vi "Create_Trajectory_Make_Trajectory.vi"(6 "TRAJECTORY_CONFIG":T1 {"MECANUM_DRIVE_KINE_CONSTRAINT"."MECA_DRIVE_KINEMATICS"."PrevCoR"."Y" format="%14.3f"; "MECANUM_DRIVE_KINE_CONSTRAINT"."MECA_DRIVE_KINEMATICS"."PrevCoR"."X" format="%14.3f"; "MECANUM_DRIVE_KINE_CONSTRAINT"."MECA_DRIVE_KINEMATICS"."RearRight"."Y" format="%14.3f"; "MECANUM_DRIVE_KINE_CONSTRAINT"."MECA_DRIVE_KINEMATICS"."RearRight"."X" format="%14.3f"; "MECANUM_DRIVE_KINE_CONSTRAINT"."MECA_DRIVE_KINEMATICS"."RearLeft"."Y" format="%14.3f"; "MECANUM_DRIVE_KINE_CONSTRAINT"."MECA_DRIVE_KINEMATICS"."RearLeft"."X" format="%14.3f"; "MECANUM_DRIVE_KINE_CONSTRAINT"."MECA_DRIVE_KINEMATICS"."FrontRight"."Y" format="%14.3f"; "MECANUM_DRIVE_KINE_CONSTRAINT"."MECA_DRIVE_KINEMATICS"."FrontRight"."X" format="%14.3f"; "MECANUM_DRIVE_KINE_CONSTRAINT"."MECA_DRIVE_KINEMATICS"."FrontLeft"."Y" format="%14.3f"; "MECANUM_DRIVE_KINE_CONSTRAINT"."MECA_DRIVE_KINEMATICS"."FrontLeft"."X" format="%14.3f"; "MECANUM_DRIVE_KINE_CONSTRAINT"."Max Speed (M/S)" format="%20.4f"; "DIFF_DRIVE_VOLTAGE_CONSTRAINT"."SIMPLE_MOTOR_FF"."Ka" format="%13.4f"; "DIFF_DRIVE_VOLTAGE_CONSTRAINT"."SIMPLE_MOTOR_FF"."Kv" format="%13.4f"; "DIFF_DRIVE_VOLTAGE_CONSTRAINT"."SIMPLE_MOTOR_FF"."Ks" format="%13.4f"; "DIFF_DRIVE_VOLTAGE_CONSTRAINT"."DIFF_DRIVE_KINEMATICS"."TrackWidth_Meters" format="%20.4f"; "DIFF_DRIVE_VOLTAGE_CONSTRAINT"."Max Voltage" format="%20.4f"; "SWERVE_DRIVE_KINE_CONSTRAINT"."SwerveKinematics"."PrevCoR"."Y" format="%14.3f"; "SWERVE_DRIVE_KINE_CONSTRAINT"."SwerveKinematics"."PrevCoR"."X" format="%14.3f"; "SWERVE_DRIVE_KINE_CONSTRAINT"."SwerveKinematics"."Modules"."Y" format="%14.3f"; "SWERVE_DRIVE_KINE_CONSTRAINT"."SwerveKinematics"."Modules"."X" format="%14.3f"; "SWERVE_DRIVE_KINE_CONSTRAINT"."Max Speed (M/S)" format="%20.4f"; "CENTRIPETAL_ACCEL_CONSTRAINT"."Max Cent Accel" format="%20.4f"; "DIFF_DRIVE_KINE_CONSTRAINT"."Max Accel (M/S2)" format="%20.4f"; "DIFF_DRIVE_KINE_CONSTRAINT"."DIFF_DRIVE_KINEMATICS"."TrackWidth_Meters" format="%20.4f"; "DIFF_DRIVE_KINE_CONSTRAINT"."Max Speed (M/S)" format="%20.4f"; "End Velocity" format="%20.4f"; "StartVelocity" format="%20.4f"; "Max Acceleration" format="%20.4f"; "MaxVelocity" format="%20.4f"}, 9 "Spline Type":enum32{"Radio Selection 1", "Radio Selection 2"}(ring), 10 "WayPoints":T13[](array[typedef]) {"WEIGHT" format="%13.3f"; "ANGLE" format="%13.3f"; "Y" format="%13.3f"; "X" format="%13.3f"}, 11 "UseWeights":bool) -> (0 "error out":errorcluster, 2 "Is Cubic":bool, 3 "TRAJECTORY":T14 {"States"."POSE"."ROTATION"."SIN" format="%13.4f"; "States"."POSE"."ROTATION"."COS" format="%13.4f"; "States"."POSE"."ROTATION"."VALUE" format="%13.4f"; "States"."POSE"."TRANSLATION"."Y" format="%14.3f"; "States"."POSE"."TRANSLATION"."X" format="%14.3f"; "TotalTImeSecs" format="%20.3f"})   [LabVIEW 2019]
uses:
  <vilib>/Rock Robotics/WPI/ThirdParty/JAS_Junk/TrajLib/TRAJECTORY.ctl
  <vilib>/Rock Robotics/WPI/ThirdParty/JAS_Junk/TrajLib/TRAJ_STATE.ctl
  <vilib>/Rock Robotics/WPI/ThirdParty/JAS_Junk/TrajLib/POSE2D.ctl
  <vilib>/Rock Robotics/WPI/ThirdParty/JAS_Junk/TrajLib/TRANSLATION2D.ctl
  <vilib>/Rock Robotics/WPI/ThirdParty/JAS_Junk/TrajLib/ROTATION2D.ctl
  <vilib>/Rock Robotics/WPI/ThirdParty/JAS_Junk/TrajLib/DISPLAY_WEIGHTED_WAYPOINT.ctl
  <vilib>/Rock Robotics/WPI/ThirdParty/JAS_Junk/TrajLib/TRAJ_CONFIG.ctl
  <vilib>/Rock Robotics/WPI/ThirdParty/JAS_Junk/TrajLib/TRAJ_CONSTRAINT_DIIF_DRIVE_KINEMATICS.ctl
  <vilib>/Rock Robotics/WPI/ThirdParty/JAS_Junk/TrajLib/DIFF_DRIVE_KINEMATICS.ctl
  <vilib>/Rock Robotics/WPI/ThirdParty/JAS_Junk/TrajLib/TRAJ_CONSTRAINT_CENTRIPETAL_ACCEL.ctl
  <vilib>/Rock Robotics/WPI/ThirdParty/JAS_Junk/TrajLib/TRAJ_CONSTRAINT_SWERVE_DRIVE_KINEMATICS.ctl
  <vilib>/Rock Robotics/WPI/ThirdParty/JAS_Junk/TrajLib/SWERVE_DRIVE_KINEMATICS.ctl
  <vilib>/Analysis/Matrix/Datatypes/RealMatrix.ctl
  <vilib>/Rock Robotics/WPI/ThirdParty/JAS_Junk/TrajLib/TRAJ_CONSTRAINT_DIIF_DRIVE_VOLTAGE.ctl
  <vilib>/Rock Robotics/WPI/ThirdParty/JAS_Junk/TrajLib/SIMPLE_MOTOR_FF.ctl
  <vilib>/Rock Robotics/WPI/ThirdParty/JAS_Junk/TrajLib/TRAJ_CONSTRAINT_MECA_DRIVE_KINEMATICS.ctl
  <vilib>/Rock Robotics/WPI/ThirdParty/JAS_Junk/TrajLib/MECA_DRIVE_KINEMATICS.ctl
  <vilib>/Rock Robotics/WPI/ThirdParty/JAS_Junk/TrajLib/Translation2d_Create.vi
  <vilib>/Rock Robotics/WPI/ThirdParty/JAS_Junk/TrajLib/Rotation2d_CreateAngle.vi
  <vilib>/Rock Robotics/WPI/ThirdParty/JAS_Junk/TrajLib/Trajectory_Library.lvlib
  <vilib>/Analysis/Matrix/NI_Matrix.lvlib
panel:
  # "ARRAY OF OTHER\nCONSTRAINTS \nGOES HERE.."
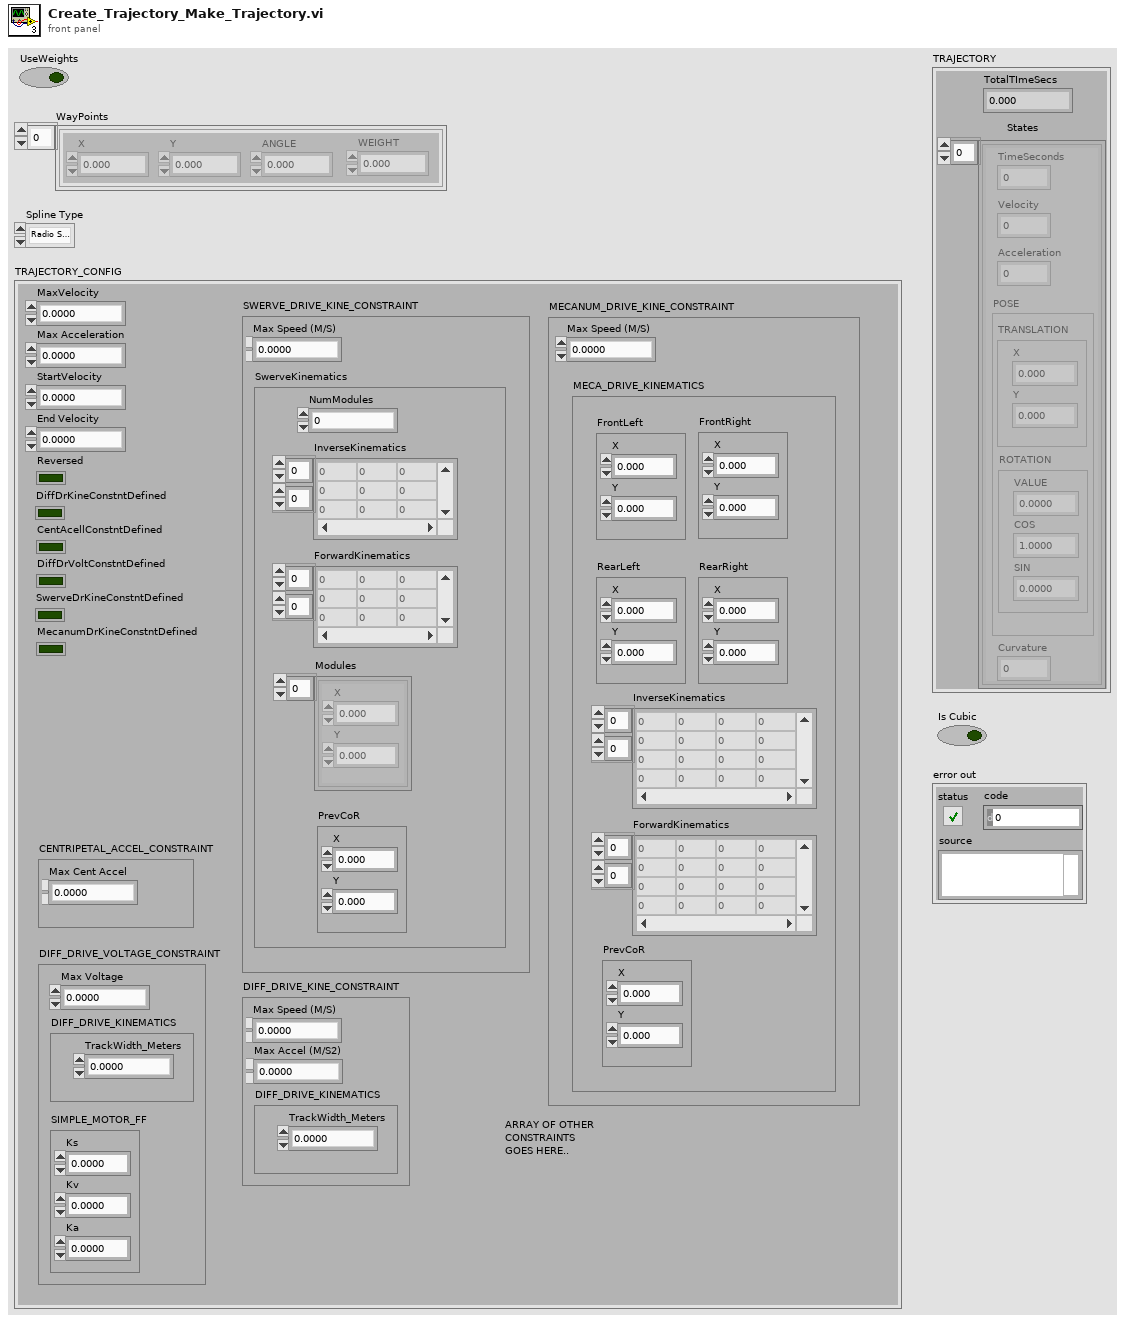
[diagram p1: front panel]
types:
  T1 = typedef "Trajectory_Library.lvlib/TRAJ_CONFIG.ctl" = cluster{"MaxVelocity":dbl, "Max Acceleration":dbl, "StartVelocity":dbl, "End Velocity":dbl, "Reversed":bool, "DiffDrKineConstntDefined":bool, "CentAcellConstntDefined":bool, "DiffDrVoltConstntDefined":bool, "DIFF_DRIVE_KINE_CONSTRAINT":T2, "CENTRIPETAL_ACCEL_CONSTRAINT":T4, "SwerveDrKineConstntDefined":bool, "SWERVE_DRIVE_KINE_CONSTRAINT":T5, "DIFF_DRIVE_VOLTAGE_CONSTRAINT":T9, "MECANUM_DRIVE_KINE_CONSTRAINT":T11, "MecanumDrKineConstntDefined":bool}
  T2 = typedef "Trajectory_Library.lvlib/TRAJ_CONSTRAINT_DIIF_DRIVE_KINEMATICS.ctl" = cluster{"Max Speed (M/S)":dbl, "DIFF_DRIVE_KINEMATICS":T3, "Max Accel (M/S2)":dbl}
  T3 = typedef "Trajectory_Library.lvlib/DIFF_DRIVE_KINEMATICS.ctl" = cluster{"TrackWidth_Meters":dbl}
  T4 = typedef "Trajectory_Library.lvlib/TRAJ_CONSTRAINT_CENTRIPETAL_ACCEL.ctl" = cluster{"Max Cent Accel":dbl}
  T5 = typedef "Trajectory_Library.lvlib/TRAJ_CONSTRAINT_SWERVE_DRIVE_KINEMATICS.ctl" = cluster{"Max Speed (M/S)":dbl, "SwerveKinematics":T6}
  T6 = typedef "Trajectory_Library.lvlib/SWERVE_DRIVE_KINEMATICS.ctl" = cluster{"NumModules":i32, "InverseKinematics":T7, "ForwardKinematics":T7, "Modules":T8[], "PrevCoR":T8}
  T7 = typedef "NI_Matrix.lvlib/RealMatrix.ctl" = dbl[][]
  T8 = typedef "Trajectory_Library.lvlib/TRANSLATION2D.ctl" = cluster{"X":dbl, "Y":dbl}
  T9 = typedef "Trajectory_Library.lvlib/TRAJ_CONSTRAINT_DIIF_DRIVE_VOLTAGE.ctl" = cluster{"Max Voltage":dbl, "DIFF_DRIVE_KINEMATICS":T3, "SIMPLE_MOTOR_FF":T10}
  T10 = typedef "Trajectory_Library.lvlib/SIMPLE_MOTOR_FF.ctl" = cluster{"Ks":dbl, "Kv":dbl, "Ka":dbl}
  T11 = typedef "Trajectory_Library.lvlib/TRAJ_CONSTRAINT_MECA_DRIVE_KINEMATICS.ctl" = cluster{"Max Speed (M/S)":dbl, "MECA_DRIVE_KINEMATICS":T12}
  T12 = typedef "Trajectory_Library.lvlib/MECA_DRIVE_KINEMATICS.ctl" = cluster{"FrontLeft":T8, "FrontRight":T8, "RearLeft":T8, "RearRight":T8, "InverseKinematics":T7, "ForwardKinematics":T7, "PrevCoR":T8}
  T13 = typedef "Trajectory_Library.lvlib/DISPLAY_WEIGHTED_WAYPOINT.ctl" = cluster{"X":dbl, "Y":dbl, "ANGLE":dbl, "WEIGHT":dbl}
  T14 = typedef "Trajectory_Library.lvlib/TRAJECTORY.ctl" = cluster{"TotalTImeSecs":dbl, "States":T15[]}
  T15 = typedef "Trajectory_Library.lvlib/TRAJ_STATE.ctl" = cluster{"TimeSeconds":dbl, "Velocity":dbl, "Acceleration":dbl, "POSE":T16, "Curvature":dbl}
  T16 = typedef "Trajectory_Library.lvlib/POSE2D.ctl" = cluster{"TRANSLATION":T8, "ROTATION":T17}
  T17 = typedef "Trajectory_Library.lvlib/ROTATION2D.ctl" = cluster{"VALUE":dbl, "COS":dbl, "SIN":dbl}
  T18 = typedef "Trajectory_Library.lvlib/WEIGHTED_WAYPOINT.ctl" = cluster{"TRANSLATION":T8, "ROTATION":T17, "SCALAR":dbl}
  T19 = typedef "Trajectory_Library.lvlib/SPLINE_CTRL_VECTOR.ctl" = cluster{"Xs":dbl[], "Ys":dbl[]}
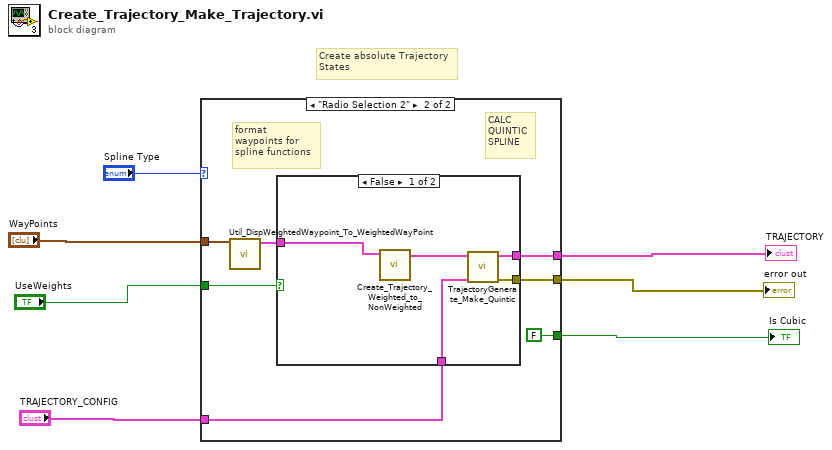
[diagram p0: block diagram]
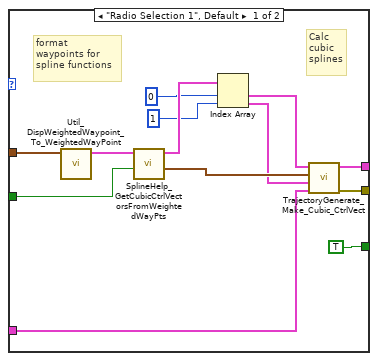
[diagram p2: hidden frame]
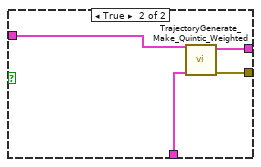
[diagram p3: hidden frame]
diagram:
  # "Create absolute Trajectory\nStates"
  n1 = case shown="\"Radio Selection 2\"" "Spline Type" {
    tunnel: [w19 w23] -> w1
    tunnel: "TRAJECTORY_CONFIG" -> [w18 w22]
    tunnel: [w20 w24] -> w7
    tunnel: [TRUE FALSE] -> w3
    tunnel: "WayPoints" -> [w16 w26]
    tunnel: "UseWeights" -> [w10 w21]
    frame "Radio Selection 1", Default {
      # "format\nwaypoints for\nspline functions"
      # "Calc\ncubic\nsplines"
      n2 = call <vilib>:"Util_DispWeightedWaypoint_To_WeightedWayPoint.vi"("DisplayWeightedWayPoints"=w16) -> ("WeightedWayPoints"=w15:T18[])  [unwired: 10 in]
      n3 = call <vilib>:"SplineHelp_GetCubicCtrlVectorsFromWeightedWayPts.vi"("Use Weights"=w10, "WeightedWayPoints"=w15) -> ("Interior WAYPOINTS"=w14:T8[], "SplineControlVectors"=w13:T19[])  [unwired: 8 in]
      n4 = Index Array(array=w13, index #1=0 ("index"), index #2=1 ("index")) -> (element #1=w12:T19, element #2=w11:T19)
      n5 = call <vilib>:"TrajectoryGenerate_Make_Cubic_CtrlVect.vi"("traj_config"=w18, "end-Spline_Ctrl_Vector"=w11, "Interior WAYPOINTS"=w14, "initial-Spline_Ctrl_Vector"=w12) -> ("error out"=w19:errorcluster, "TRAJECTORY"=w20:T14)  [unwired: 6 in]
    }
    frame "Radio Selection 2" {
      # "format\nwaypoints for\nspline functions"
      # "CALC\nQUINTIC\nSPLINE"
      n6 = call <vilib>:"Util_DispWeightedWaypoint_To_WeightedWayPoint.vi"("DisplayWeightedWayPoints"=w26) -> ("WeightedWayPoints"=w25:T18[])  [unwired: 10 in]
      n7 = case shown="False" w21 {
        tunnel: [w32 w36] -> w24
        tunnel: [w31 w35] -> w23
        tunnel: w25 -> [w28 w34]
        tunnel: w22 -> [w29 w33]
        frame False {
          n8 = call "Create_Trajectory_Weighted_to_NonWeighted.vi"("WeightedWayPoints"=w28) -> ("WayPoints"=w30:T16[])  [unwired: 10 in]
          n9 = call <vilib>:"TrajectoryGenerate_Make_Quintic.vi"("traj_config"=w29, "waypointPOSE"=w30) -> ("error out"=w31:errorcluster, "TRAJECTORY"=w32:T14)  [unwired: 8 in]
        }
        frame True {
          n10 = call <vilib>:"TrajectoryGenerate_Make_Quintic_Weighted.vi"("traj_config"=w33, "WeightedWaypointPOSE"=w34) -> ("error out"=w35:errorcluster, "TRAJECTORY"=w36:T14)  [unwired: 8 in]
        }
      }
    }
  }
  "TRAJECTORY" <- w7
  "Is Cubic" <- w3
  "error out" <- w1
